vi "Solve2.vi"(8 "Error In":errorcluster, 11 "object in":refnum<class "2022_8.lvclass">) -> (0 "Error Out":errorcluster, 2 "Result":u64, 3 "object out":refnum<class "2022_8.lvclass">)   [LabVIEW 2020, in "2022_8.lvclass"]
uses:
  2022_8.lvclass
  2022_8.lvclass/2022_8.ctl
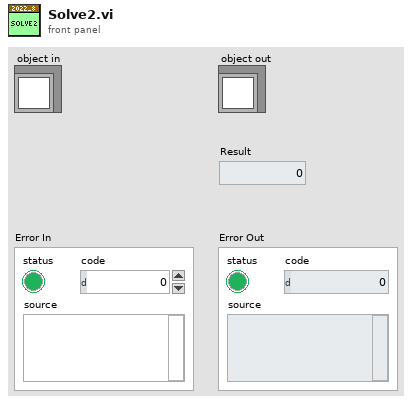
[diagram p1: front panel]
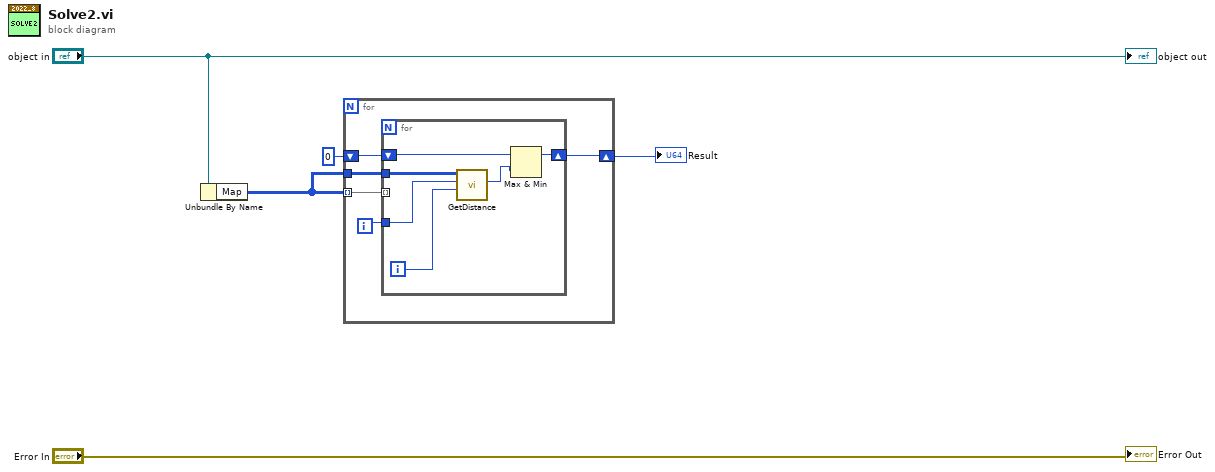
[diagram p0: block diagram]
diagram:
  n1 = Unbundle By Name("object in") -> ("Map"=w3:u8[][])
  n2 = for {
    tunnel: w3 -> [w10] mode=indexing
    tunnel: w3 -> [w9]
    shift-right: [w7] -> w1
    shift-left: 0 -> [w6]
    i -> [w8]
    n3 = for {
      tunnel: w10 -> [_] mode=indexing
      tunnel: w9 -> [w16]
      tunnel: w8 -> [w15]
      shift-right: [w12] -> w7
      shift-left: w6 -> [w11]
      i -> [w14]
      n4 = call "GetDistance.vi"("Column"=w14, "Row"=w15, "MapIn"=w16) -> ("Score"=w13:i32)  [unwired: 8 in]
      n5 = Max & Min(x=w11, y=w13) -> (max(x,y)=w12:i32)  [unwired: 1 out]
    }
  }
  "Result" <- w1
  "Error Out" <- "Error In"
  "object out" <- "object in"
